vi "Trav_Prog_Extra_Commands.vi"() -> (1 "Extra Commands Array":string[](array[string]), 2 "Argument Examples":string[](array[string]))   [LabVIEW 2022 SP3]
uses:
  Globals/Extra_Commands_Global.vi
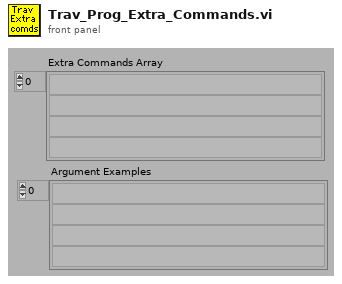
[diagram p1: front panel]
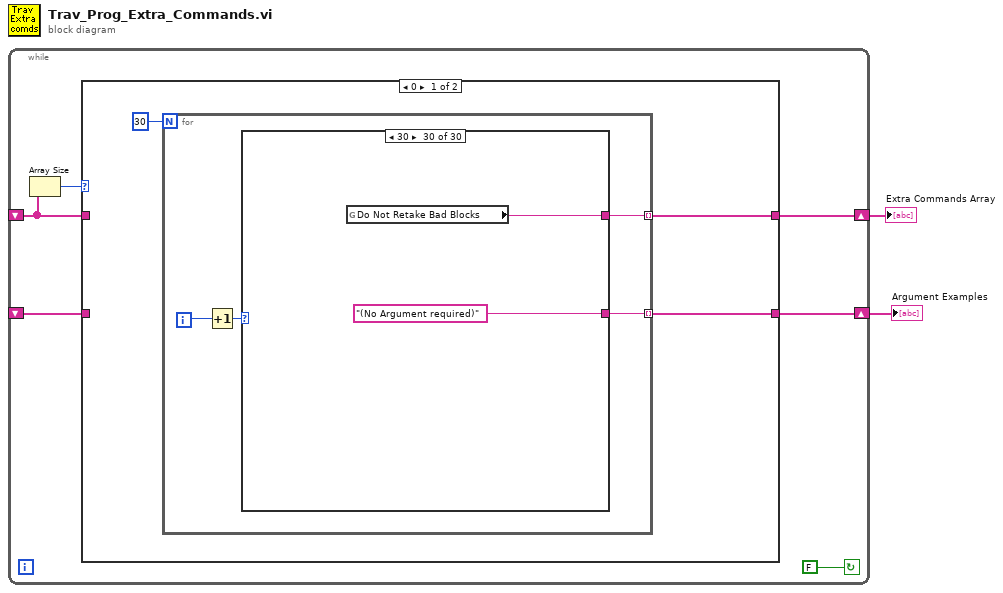
[diagram p0: block diagram]
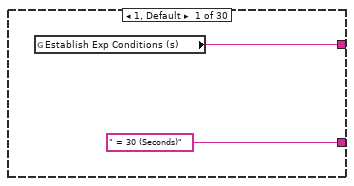
[diagram p2: hidden frame]
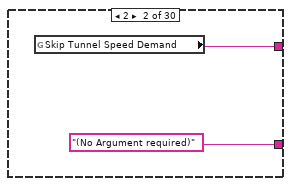
[diagram p3: hidden frame]
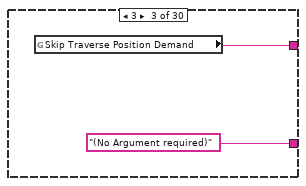
[diagram p4: hidden frame]
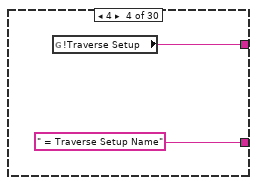
[diagram p5: hidden frame]
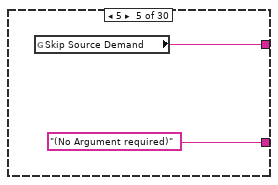
[diagram p6: hidden frame]
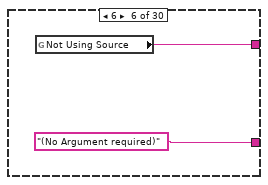
[diagram p7: hidden frame]
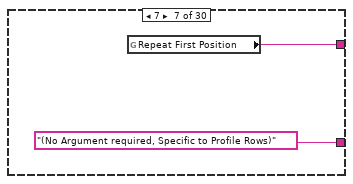
[diagram p8: hidden frame]
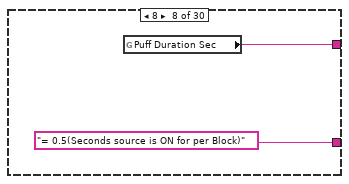
[diagram p9: hidden frame]
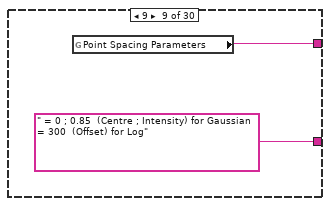
[diagram p10: hidden frame]
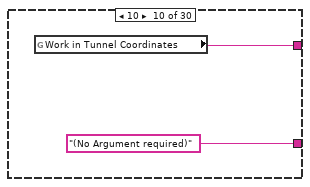
[diagram p11: hidden frame]
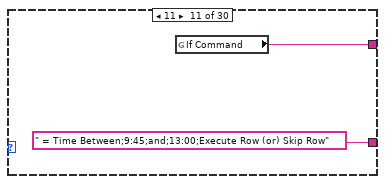
[diagram p12: hidden frame]
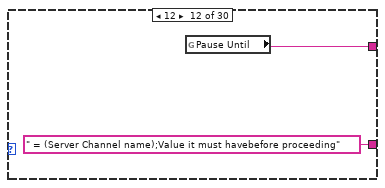
[diagram p13: hidden frame]
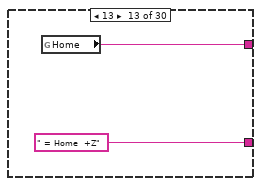
[diagram p14: hidden frame]
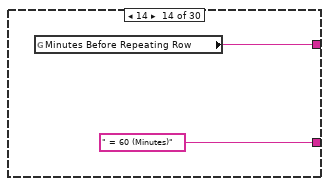
[diagram p15: hidden frame]
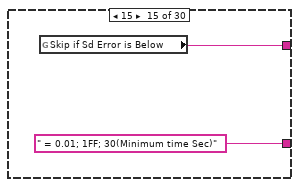
[diagram p16: hidden frame]
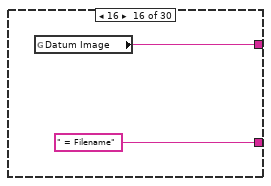
[diagram p17: hidden frame]
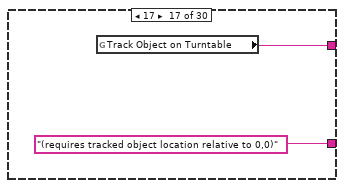
[diagram p18: hidden frame]
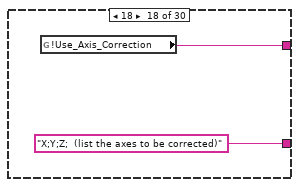
[diagram p19: hidden frame]
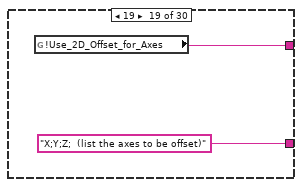
[diagram p20: hidden frame]
diagram:
  n1 = while {
    shift-left: _ -> [w4]
    shift-right: [w7] -> w1
    shift-left: _ -> [w5]
    shift-right: [w8] -> w2
    stop <- FALSE continue-if-true
    n2 = Array Size(array=w5) -> (size(s)=w6:i32)
    n3 = case shown="0" w6 {
      tunnel: [w10 w77] -> w8
      tunnel: [w9 w76] -> w7
      tunnel: w5 -> [_ w77]
      tunnel: w4 -> [_ w76]
      frame 0 {
        n4 = for {
          N: 30 -> [_]
          tunnel: [w13] -> w10 mode=indexing
          tunnel: [w12] -> w9 mode=indexing
          i -> [w15]
          n5 = Increment(x=w15) -> (x+1=w14:i32)
          n6 = case shown="30" w14 {
            tunnel: [w17 w19 w21 w23 w25 w27 w29 w31 w33 w35 w37 w39 w41 w43 w45 w47 w49 w51 w53 w55 w57 w59 w61 w63 w65 w67 w69 w71 w73 w75] -> w13
            tunnel: [" = 30 (Seconds)" "(No Argument required)" "(No Argument required)" " = Traverse Setup Name" "(No Argument required)" "(No Argument required)" "(No Argument required, Specific to Profile Rows)" "= 0.5(Seconds source is ON for per Block)" " = 0 ; 0.85  (Centre ; Intensity) for Gaussian = 300  (Offset) for Log" "(No Argument required)" " = Time Between;9:45;and;13:00;Execute Row (or) Skip Row" " = (Server Channel name);Value it must havebefore proceeding" " = Home  +Z" " = 60 (Minutes)" " = 0.01; 1FF; 30(Minimum time Sec)" " = Filename" "(requires tracked object location relative to 0,0)" "X;Y;Z;  (list the axes to be corrected)" "X;Y;Z;  (list the axes to be offset)" "Name of Plug_In" "(No Argument required)" "(No Argument required)" "1; -1; 0 (list dx;dy;dz)" "1; -1; 0 (list dx;dy;dz)" "10" " = GMU1 Source" "(No Argument required)" "0.1" "(No Argument required)" "(No Argument required)"] -> w12
            frame 1, Default {
              n7 = global read "Extra_Commands_Global.vi" "Establish Exp Conditions (s)"() -> (w17:string)
            }
            frame 2 {
              n8 = global read "Extra_Commands_Global.vi" "Skip Tunnel Speed Demand"() -> (w19:string)
            }
            frame 3 {
              n9 = global read "Extra_Commands_Global.vi" "Skip Traverse Position Demand"() -> (w21:string)
            }
            frame 4 {
              n10 = global read "Extra_Commands_Global.vi" "!Traverse Setup"() -> (w23:string)
            }
            frame 5 {
              n11 = global read "Extra_Commands_Global.vi" "Skip Source Demand"() -> (w25:string)
            }
            frame 6 {
              n12 = global read "Extra_Commands_Global.vi" "Not Using Source"() -> (w27:string)
            }
            frame 7 {
              n13 = global read "Extra_Commands_Global.vi" "Repeat First Position"() -> (w29:string)
            }
            frame 8 {
              n14 = global read "Extra_Commands_Global.vi" "Puff Duration Sec"() -> (w31:string)
            }
            frame 9 {
              n15 = global read "Extra_Commands_Global.vi" "Point Spacing Parameters"() -> (w33:string)
            }
            frame 10 {
              n16 = global read "Extra_Commands_Global.vi" "Work in Tunnel Coordinates"() -> (w35:string)
            }
            frame 11 {
              n17 = global read "Extra_Commands_Global.vi" "If Command"() -> (w37:string)
            }
            frame 12 {
              n18 = global read "Extra_Commands_Global.vi" "Pause Until"() -> (w39:string)
            }
            frame 13 {
              n19 = global read "Extra_Commands_Global.vi" "Home"() -> (w41:string)
            }
            frame 14 {
              n20 = global read "Extra_Commands_Global.vi" "Minutes Before Repeating Row"() -> (w43:string)
            }
            frame 15 {
              n21 = global read "Extra_Commands_Global.vi" "Skip if Sd Error is Below"() -> (w45:string)
            }
            frame 16 {
              n22 = global read "Extra_Commands_Global.vi" "Datum Image"() -> (w47:string)
            }
            frame 17 {
              n23 = global read "Extra_Commands_Global.vi" "Track Object on Turntable"() -> (w49:string)
            }
            frame 18 {
              n24 = global read "Extra_Commands_Global.vi" "!Use_Axis_Correction"() -> (w51:string)
            }
            frame 19 {
              n25 = global read "Extra_Commands_Global.vi" "!Use_2D_Offset_for_Axes"() -> (w53:string)
            }
            frame 20 {
              n26 = global read "Extra_Commands_Global.vi" "Trav_Profile_Plug_In"() -> (w55:string)
            }
            frame 21 {
              n27 = global read "Extra_Commands_Global.vi" "Suppress Route Check Errors"() -> (w57:string)
            }
            frame 22 {
              n28 = global read "Extra_Commands_Global.vi" "!3D Live Position Offset"() -> (w59:string)
            }
            frame 23 {
              n29 = global read "Extra_Commands_Global.vi" "!Offset dx;dy;dz in Tunnel Coord"() -> (w61:string)
            }
            frame 24 {
              n30 = global read "Extra_Commands_Global.vi" "!Offset dx;dy;dz in Model Coord"() -> (w63:string)
            }
            frame 25 {
              n31 = global read "Extra_Commands_Global.vi" "Block Length (s)"() -> (w65:string)
            }
            frame 26 {
              n32 = global read "Extra_Commands_Global.vi" "Gas Line Name"() -> (w67:string)
            }
            frame 27 {
              n33 = global read "Extra_Commands_Global.vi" "sortPoints"() -> (w69:string)
            }
            frame 28 {
              n34 = global read "Extra_Commands_Global.vi" "!Traverse Speed Factor"() -> (w71:string)
            }
            frame 29 {
              n35 = global read "Extra_Commands_Global.vi" "Skip Source Establishment"() -> (w73:string)
            }
            frame 30 {
              n36 = global read "Extra_Commands_Global.vi" "Do Not Retake Bad Blocks"() -> (w75:string)
            }
          }
        }
      }
      frame 1, Default {
      }
    }
  }
  "Extra Commands Array" <- w2
  "Argument Examples" <- w1
